vi "AnimExecGen.vi"(8 "ErrorIn(No Error)":errorcluster caption="entrée d'erreur (pas d'erreur)", 10 "Animer l'exécution ?":bool, 11 "ViRef":refnum<vi>) -> (0 "sortie d'erreur":errorcluster)   [LabVIEW 2010]
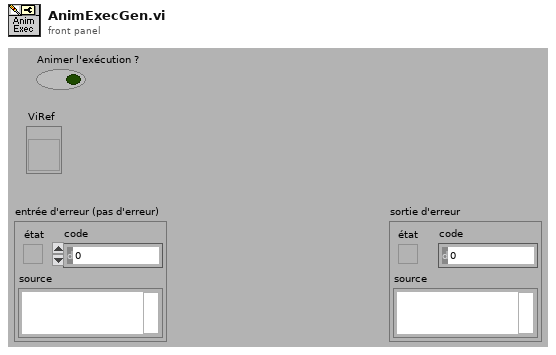
[diagram p1: front panel]
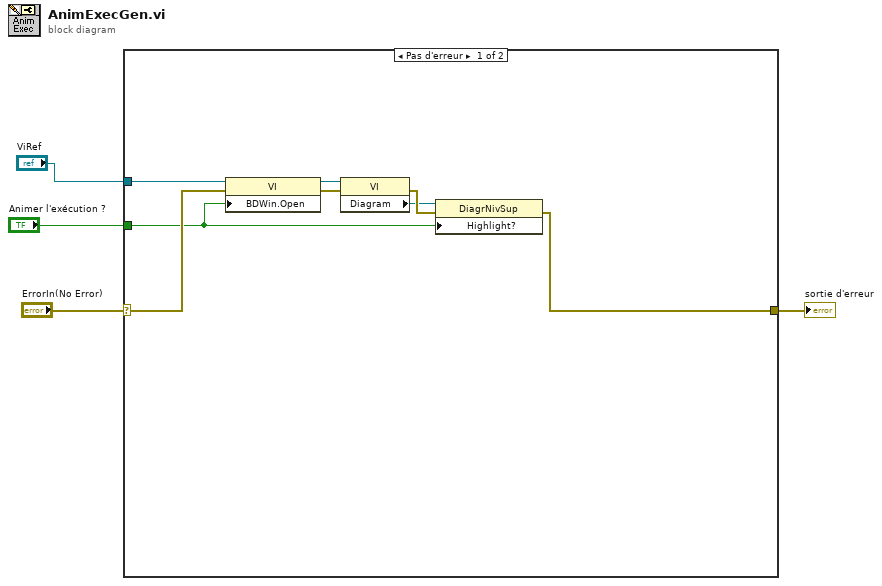
[diagram p0: block diagram]
diagram:
  n1 = case shown="Pas d'erreur" "ErrorIn(No Error)" {
    selector: "ErrorIn(No Error)" -> [w7 w13]
    tunnel: [w11 w13] -> w3
    tunnel: "ViRef" -> [w9 _]
    tunnel: "Animer l'exécution ?" -> [w5 _]
    frame No Error {
      n2 = property class="VI"(reference=w9, error in=w7, "BDWin.Open"=w5) -> (reference out=w8:refnum<vi>, error out=w6:errorcluster)
      n3 = property class="VI"(reference=w8, error in=w6) -> (error out=w12:errorcluster, "Diagram"=w10:refnum<vi>)  [unwired: 1 out]
      n4 = property class="DiagrNivSup"(reference=w10, error in=w12, "Highlight?"=w5) -> (error out=w11:errorcluster)  [unwired: 1 out]
    }
    frame Error {
    }
  }
  "sortie d'erreur" <- w3
